vi "Folder Dialog.vi"(8 "error in":errorcluster) -> (0 "error out":errorcluster, 2 "ButtonPressed":i32(ring) items=["None", "OK", "Cancel", "Abort", "Retry", "Ignore", "Yes", "No"], 3 "Path":path)   [LabVIEW 2019, in "GUI.lvlib"]
uses:
  GUI.lvlib
  System.Windows.Forms
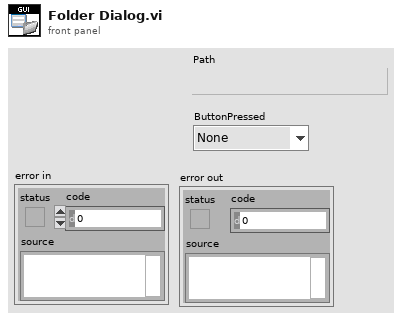
[diagram p1: front panel]
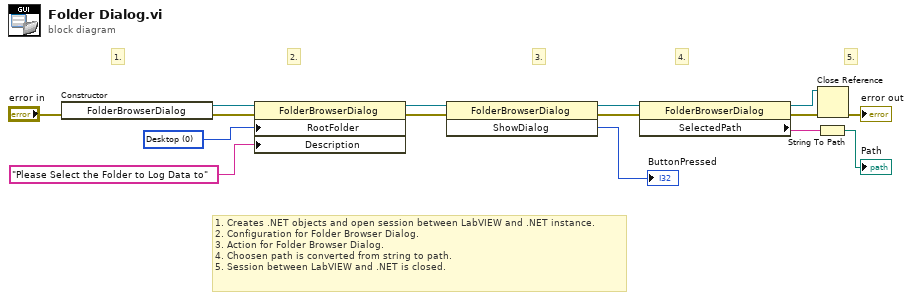
[diagram p0: block diagram]
diagram:
  w13 = 0 items=["Desktop"=0, "Programs"=2, "Personal, MyDocuments"=5, "Favorites"=6, "Startup"=7, "Recent"=8, "SendTo"=9, "StartMenu"=11, "MyMusic"=13, "DesktopDirectory"=16, "MyComputer"=17, "Templates"=21, "ApplicationData"=26, "LocalApplicationData"=28, "InternetCache"=32, "Cookies"=33, "History"=34, "CommonApplicationData"=35, "System"=37, "ProgramFiles"=38, "MyPictures"=39, "CommonProgramFiles"=43] ("RootFolder")
  # "1. Creates .NET objects and open session between LabVIEW and .NET instance.\n2. Configuration for Folder Browser Dialog.\n3. Action for Folder Browser Dialog.\n4. Choosen path is converted from string to path.\n5. Session between LabVIEW and .NET is closed."
  # "5."
  # "4."
  # "3."
  # "2."
  # "1."
  n1 = constructor class="FolderBrowserDialog"(error in="error in") -> (reference out=w15:refnum<k24>, error out=w14:errorcluster)  [unwired: 2 in, 1 out]
  n2 = property class="FolderBrowserDialog"(reference=w15, error in=w14, "RootFolder"=w13, "Description"="Please Select the Folder to Log Data to") -> (reference out=w11:refnum<k24>, error out=w10:errorcluster)
  n3 = invoke class="FolderBrowserDialog" method="ShowDialog"(reference=w11, error in=w10) -> (reference out=w9:refnum<k24>, error out=w8:errorcluster, "ShowDialog"=→"ButtonPressed":i32)  [unwired: 1 in]
  n4 = property class="FolderBrowserDialog"(reference=w9, error in=w8) -> (reference out=w5:refnum<k24>, error out=w6:errorcluster, "SelectedPath"=w7:string)
  n5 = String To Path(string=w7) -> (path=→"Path":path)
  n6 = Close Reference(reference=w5, error in (no error)=w6) -> (error out=→"error out":errorcluster)
